vi "Draw Exponential.vi"(8 "B":dbl, 9 "A":dbl, 10 "tau":dbl, 11 "time":dbl[](array[numeric])) -> (3 "ExponentialOut":dbl[](array[numeric]))   [LabVIEW 2014, in "Exponential Fit Library.lvlib" / "Fit Exponential.lvclass"]
uses:
  Fit Exponential.lvclass
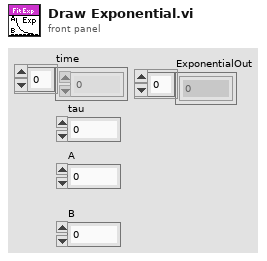
[diagram p1: front panel]
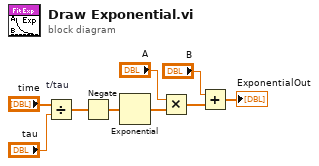
[diagram p0: block diagram]
diagram:
  n1 = Divide "t/tau"(x="time", y="tau") -> (x/y=w4:dbl[])
  n2 = Negate(x=w4) -> (-x=w3:dbl[])
  n3 = Exponential(1:w3) -> (0:w9:dbl[])
  n4 = Multiply(x="A", y=w9) -> (x*y=w7:dbl[])
  n5 = Add(x="B", y=w7) -> (x+y=→"ExponentialOut":dbl[])
